vi "FG Status Indicators.vi"(2 "FG Action (Read)":T2, 3 "Status Indicators in":T1) -> (1 "Status Indicators out":T1)   [LabVIEW 2009]
uses:
  Actions for FG's.ctl
  Status Indicators.ctl
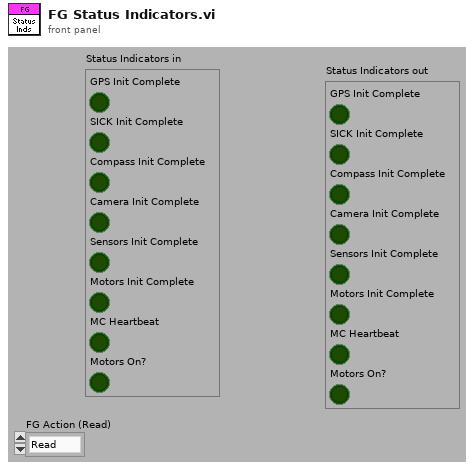
[diagram p1: front panel]
types:
  T1 = typedef "Status Indicators.ctl" = cluster{"GPS Init Complete":bool, "SICK Init Complete":bool, "Compass Init Complete":bool, "Camera Init Complete":bool, "Sensors Init Complete":bool, "Motors Init Complete":bool, "MC Heartbeat":bool, "Motors On?":bool}
  T2 = typedef "Actions for FG's.ctl" = enum16{"Read", "Write"}
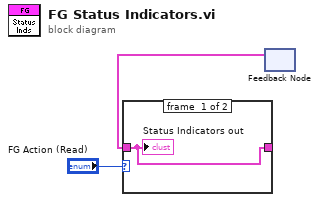
[diagram p0: block diagram]
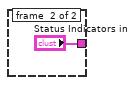
[diagram p2: hidden frame]
diagram:
  n1 = feedback #1() -> (w1:T1)  [unwired: 1 in]
  n2 = case shown="\"Write\"" "FG Action (Read)" {
    tunnel: [w4 "Status Indicators in"] -> w2
    tunnel: w1 -> [w4 _]
    frame #0 {
      "Status Indicators out" <- w4
    }
    frame #1 {
    }
  }
